vi "Create-Delete Link.vi"(5 "Username":string, 6 "Password":string, 7 "Address":string, 8 "Error In":errorcluster) -> (0 "Error Out":errorcluster)   [LabVIEW 2018, in "Tests.lvlib" / "SFTP.lvlib"]
uses:
  SFTP.lvlib
  src/Toolkit/SFTP Attributes/Type Definitions/File Types.ctl
  src/Toolkit/SFTP Attributes/SFTP Attributes.lvclass/SFTP Attributes.ctl
  src/Toolkit/SSH/SSH.lvclass/SSH.ctl
  src/Toolkit/SSH/Utility/Read Shared Library.vi
  src/Toolkit/SFTP Attributes/Support/Create from SFTP.vi
  src/Toolkit/Support/Check Status.vi
  src/Toolkit/SFTP Attributes/Support/Destroy to SFTP.vi
  <vilib>/addons/_JKI Toolkits/Caraya/classes/Test/Test.lvclass
  <vilib>/addons/_JKI Toolkits/Caraya/classes/Assert/Assert.lvclass
  src/Toolkit/SFTP/SFTP.lvclass
  src/Toolkit/SFTP Attributes/SFTP Attributes.lvclass
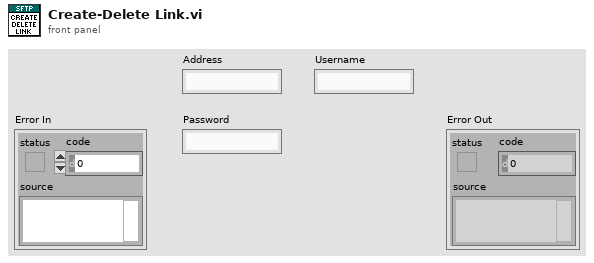
[diagram p1: front panel]
types:
  T1 = typedef "Toolkit.lvlib/SFTP Attributes.lvclass/File Types.ctl" = u32
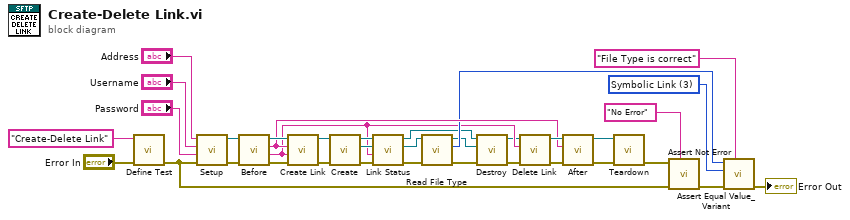
[diagram p0: block diagram]
diagram:
  w14 = T1 3 items=["Regular"=1, "Directory"=2, "Symbolic Link"=3, "Special"=4, "Unknown"=5, "Socket"=6, "Character Device"=7, "Block Device"=8, "FIFO"=9] ("File Type")
  n1 = call <vilib>:"Define Test.vi"("error in (no error)"="Error In", "Label (VI Title)"="Create-Delete Link") -> ("error out"=w30:errorcluster)  [unwired: 9 in]
  n2 = call "Setup.vi"("Error In"=w30, "Password"="Password", "Username"="Username", "Address"="Address") -> ("Error Out"=w31:errorcluster, "Sesssion"=w26:refnum<class "Session.lvclass">)  [unwired: 6 in]
  n3 = call "Before.vi"("Error In"=w31, "Session In"=w26) -> ("Error Out"=w21:errorcluster, "Remote Link Path"=w8:string, "Remote Source Path"=w18:string, "SFTP Out"=w22:refnum<class "SFTP.lvclass">)  [unwired: 6 in]
  n4 = call "Create Link.vi"("Error In"=w21, "Remote Link Path"=w8, "Remote Source Path"=w18, "SFTP In"=w22) -> ("Error Out"=w9:errorcluster, "SFTP Out"=w13:refnum<class "SFTP.lvclass">)  [unwired: 6 in]
  n5 = call-poly "Create.vi"("Error In"=w9, "SFTP In"=w13) -> ("Error Out"=w10:errorcluster, "SFTP Attributes"=w11:refnum<class "SFTP Attributes.lvclass">, "SFTP Out"=w12:refnum<class "SFTP.lvclass">)  [unwired: 7 in]
  n6 = call "Link Status.vi"("Error In"=w10, "Remote Path"=w8, "Attributes In"=w11, "SFTP In"=w12) -> ("Error Out"=w7:errorcluster, "Attributes Out"=w6:refnum<class "SFTP Attributes.lvclass">, "SFTP Out"=w4:refnum<class "SFTP.lvclass">)  [unwired: 5 in]
  n7 = call "Read File Type.vi"("Error In"=w7, "SFTP Attributes In"=w6) -> ("Error Out"=w5:errorcluster, "File Type"=w15:T1, "SFTP Attributes Out"=w3:refnum<class "SFTP Attributes.lvclass">)  [unwired: 7 in]
  n8 = call-poly "Destroy.vi"("Error In"=w5, "SFTP Attributes"=w3, "SFTP In"=w4) -> ("Error Out"=w1:errorcluster, "SFTP Out"=w2:refnum<class "SFTP.lvclass">)  [unwired: 7 in]
  n9 = call "Delete Link.vi"("Error In"=w1, "Remote Path"=w8, "SFTP In"=w2) -> ("Error Out"=w19:errorcluster, "SFTP Out"=w20:refnum<class "SFTP.lvclass">)  [unwired: 7 in]
  n10 = call "After.vi"("Error In"=w19, "Remote Source Path"=w18, "SFTP In"=w20) -> ("Error Out"=w25:errorcluster, "Session Out"=w23:refnum<class "Session.lvclass">)  [unwired: 7 in]
  n11 = call "Teardown.vi"("Error In"=w25, "Session"=w23) -> ("Error Out"=w24:errorcluster)  [unwired: 9 in]
  n12 = call <vilib>:"Assert Not Error.vi"("Label"="No Error", "error in (no error)"=w30, "Not Error?"=w24) -> ("error out"=w32:errorcluster)  [unwired: 8 in]
  n13 = call <vilib>:"Assert Equal Value_Variant.vi"("Label"="File Type is correct", "error in (no error)"=w32, "Y"=w14, "X"=w15) -> ("error out"=→"Error Out":errorcluster)  [unwired: 7 in]
